vi "DOConfigTrigger.vi"(0 "object in":refnum<class "AD2_DO_SDK.lvclass">, 5 "error in (no error)":errorcluster) -> (14 "object out":refnum<class "AD2_DO_SDK.lvclass">, 19 "error out":errorcluster)   [LabVIEW 2021, in "AD2_DO_SDK.lvclass"]
uses:
  AD2_DO_SDK.lvclass
  AD2_DO_SDK.lvclass/AD2_DO_SDK.ctl
  Olasdwf/Olasdwf.lvlib
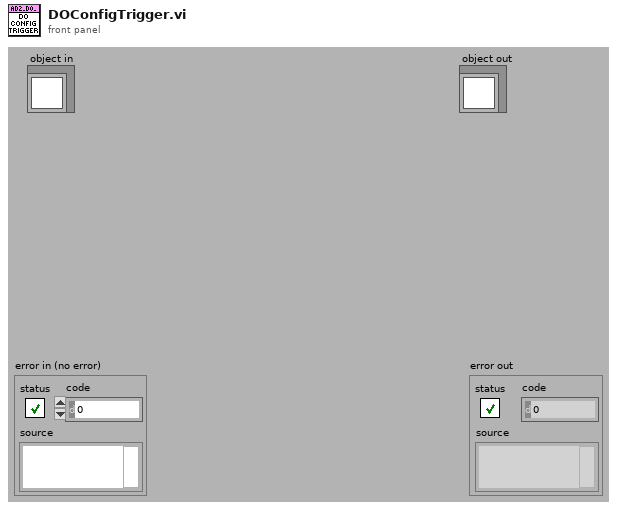
[diagram p1: front panel]
types:
  T1 = typedef "AD2_SDK.lvclass/AD2TriggerSources.ctl" = enum8{"trigrsrcNone", "trigsrcPC", "trigsrcDetectorAnalogIn", "trigsrcDetectorDigitalIn", "trigsrcAnalogIn", "trigsrcDigitalIn", "trigsrcDigitalOut", "trigsrcAnalogOut1", "trigsrcAnalogOut2", "trigsrcAnalogOut3", "trigsrcAnalogOut4", "trigsrcExternal1", "trigsrcExternal2", "trigsrcExternal3", "trigsrcExternal4", ""}
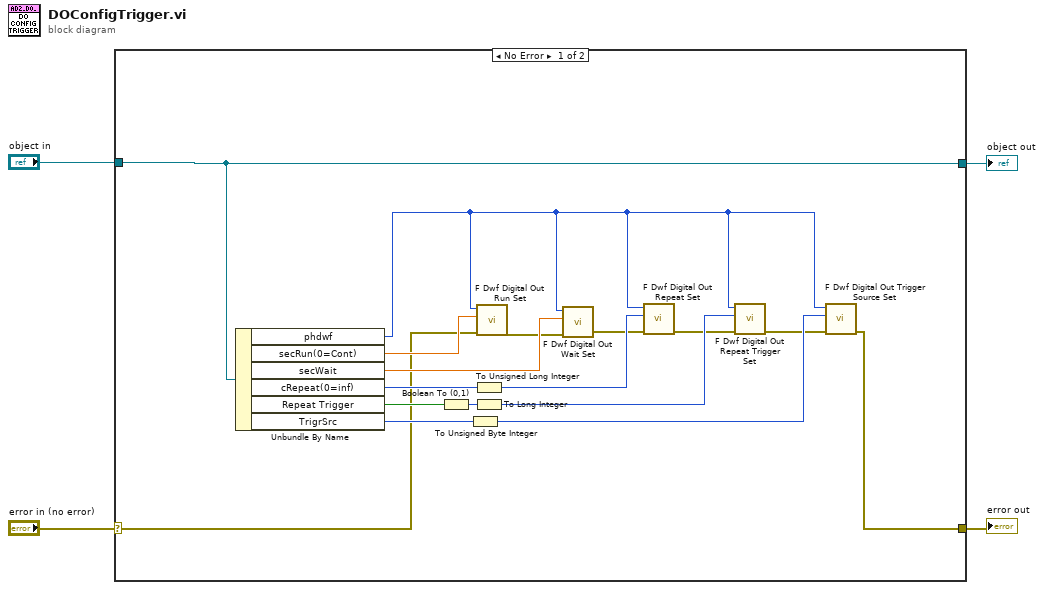
[diagram p0: block diagram]
diagram:
  n1 = case shown="No Error" "error in (no error)" {
    selector: "error in (no error)" -> [w7 w23]
    tunnel: [w6 w23] -> w3
    tunnel: [w5 w22] -> w1
    tunnel: "object in" -> [w5 w22]
    frame No Error {
      n2 = Unbundle By Name(w5) -> ("phdwf"=w12:i32, "secRun(0=Cont)"=w21:dbl, "secWait"=w20:dbl, "cRepeat(0=inf)"=w19:i32, "Repeat Trigger"=w15:bool, "TrigrSrc"=w14:T1)
      n3 = Boolean To (0,1)(Boolean=w15) -> (0, 1=w16:i16)
      n4 = To Unsigned Byte Integer(number=w14) -> (unsigned 8bit integer=w13:u8)
      n5 = To Unsigned Long Integer(number=w19) -> (unsigned 32bit integer=w18:u32)
      n6 = To Long Integer(number=w16) -> (32bit integer=w17:i32)
      n7 = call "F Dwf Digital Out Run Set.vi"("error in (no error)"=w7, "secRun"=w21, "hdwf"=w12) -> ("error out"=w8:errorcluster)  [unwired: 7 in, 1 out]
      n8 = call "F Dwf Digital Out Wait Set.vi"("error in (no error)"=w8, "secWait"=w20, "hdwf"=w12) -> ("error out"=w9:errorcluster)  [unwired: 7 in, 1 out]
      n9 = call "F Dwf Digital Out Repeat Set.vi"("error in (no error)"=w9, "cRepeat"=w18, "hdwf"=w12) -> ("error out"=w10:errorcluster)  [unwired: 7 in, 1 out]
      n10 = call "F Dwf Digital Out Repeat Trigger Set.vi"("error in (no error)"=w10, "fRepeatTrigger"=w17, "hdwf"=w12) -> ("error out"=w11:errorcluster)  [unwired: 7 in, 1 out]
      n11 = call "F Dwf Digital Out Trigger Source Set.vi"("error in (no error)"=w11, "trigsrc"=w13, "hdwf"=w12) -> ("error out"=w6:errorcluster)  [unwired: 7 in, 1 out]
    }
    frame Error {
    }
  }
  "error out" <- w3
  "object out" <- w1
